vi "HttpGet.vi"(6 "request specific headers":T1[](array[typedef]), 8 "error in":errorcluster, 10 "url":string, 11 "reQwestClient in":refnum<class "reQwestClient.lvclass">) -> (0 "error out":errorcluster, 1 "headers":cluster{"name":string, "value":string}[](array[cluster]), 2 "response_body":string, 3 "reQwestClient out":refnum<class "reQwestClient.lvclass">)   [LabVIEW 2020, in "reQwestClient.lvclass"]
uses:
  reQwestClient.lvclass
  <vilib>/addons/_JKI.lib/REST Client/classes/REST Client/HTTP Header.ctl
  submodules/reqwest-rs-labview/lv_src/Types/http_method_enum.ctl
  reQwestClient.lvclass/reQwestClient.ctl
  submodules/reqwest-rs-labview/lv_src/Request/Request.lvclass
  submodules/reqwest-rs-labview/lv_src/Client/Client.lvclass
  submodules/reqwest-rs-labview/lv_src/reqwest.lvlib
  submodules/reqwest-rs-labview/lv_src/RequestBuilder/RequestBuilder.lvclass
  submodules/reqwest-rs-labview/lv_src/Headers/Headers.lvclass
  <vilib>/addons/_JKI.lib/REST Client/classes/REST Client/REST Client.lvclass
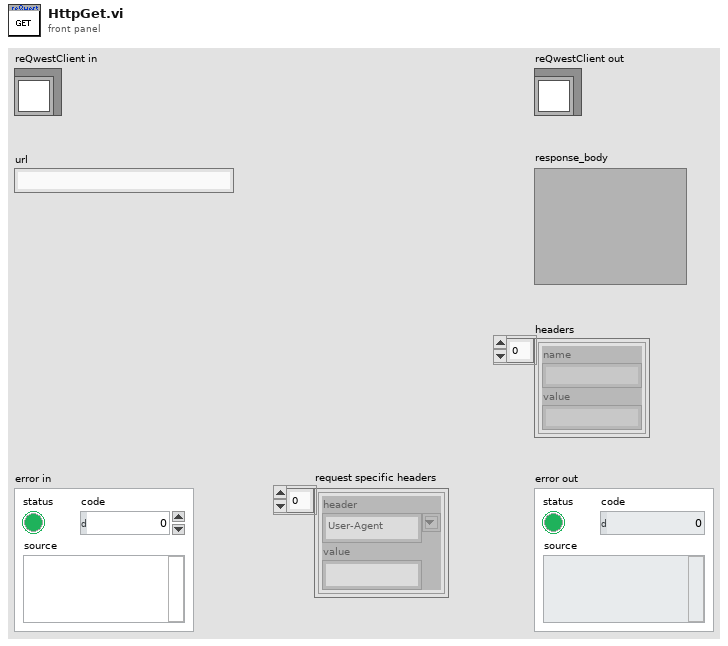
[diagram p1: front panel]
types:
  T1 = typedef "REST Client.lvlib/REST Client.lvclass/HTTP Header.ctl" = cluster{"header":string, "value":string}
  T2 = typedef "reqwest.lvlib/http_method_enum.ctl" = enum8{"<select>", "GET", "POST", "PUT", "DELETE", "HEAD", "OPTIONS", "CONNECT", "PATCH", "TRACE"}
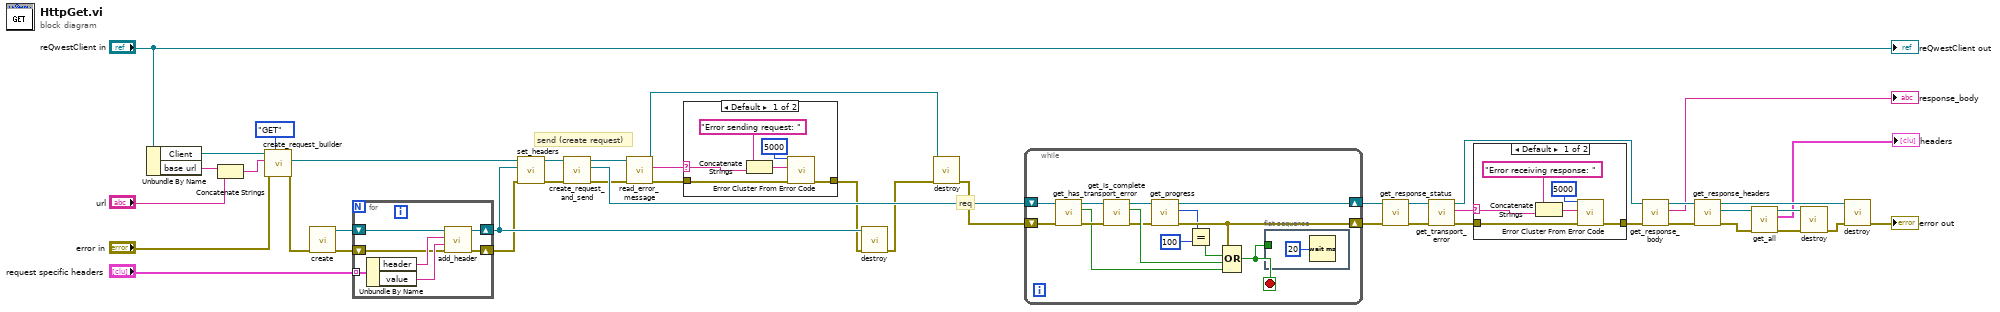
[diagram p0: block diagram]
diagram:
  # "send (create request)"
  # "req"
  n1 = Unbundle By Name("reQwestClient in") -> ("Client"=w25:refnum<class "Client.lvclass">, "base url"=w11:string)
  n2 = Concatenate Strings(w11, "url") -> (w9:string)
  n3 = call "create_request_builder.vi"("HTTP Method"=http_method_enum."GET", "error in (no error)"="error in", "url"=w9, "Client in"=w25) -> ("error out"=w15:errorcluster, "RequestBuilder out"=w21:refnum<class "RequestBuilder.lvclass">)  [unwired: 5 in, 1 out]
  n4 = call "create.vi"("error in (no error)"=w15) -> ("error out"=w22:errorcluster, "Headers out"=w24:refnum<class "Headers.lvclass">)  [unwired: 9 in]
  n5 = for {
    tunnel: "request specific headers" -> [w50] mode=indexing
    shift-right: [w46] -> w18
    shift-left: w24 -> [w51]
    shift-right: [w45] -> w16
    shift-left: w22 -> [w47]
    n6 = Unbundle By Name(w50) -> ("header"=w49:string, "value"=w48:string)
    n7 = call "add_header.vi"("error in (no error)"=w47, "value"=w48, "key"=w49, "Headers in"=w51) -> ("error out"=w45:errorcluster, "Headers out"=w46:refnum<class "Headers.lvclass">)  [unwired: 5 in, 1 out]
  }
  n8 = call "set_headers.vi"("error in (no error)"=w16, "Headers"=w18, "obj in"=w21) -> ("error out"=w19:errorcluster, "obj out"=w20:refnum<class "RequestBuilder.lvclass">)  [unwired: 6 in, 1 out]
  n9 = call "create_request_and_send.vi"("error in"=w19, "obj in"=w20) -> ("error out"=w28:errorcluster, "request"=w31:refnum<class "Request.lvclass">, "obj out"=w29:refnum<class "RequestBuilder.lvclass">)  [unwired: 7 in]
  n10 = call "read_error_message.vi"("error in (no error)"=w28, "RequestBuilder in"=w29) -> ("error out"=w8:errorcluster, "error_message"=w6:string, "RequestBuilder in"=w30:refnum<class "RequestBuilder.lvclass">)  [unwired: 7 in]
  n11 = case shown="Default" w6 {
    selector: w6 -> [w54 _]
    tunnel: w8 -> [w57 w58]
    tunnel: [w56 w58] -> w7
    frame Default {
      n12 = Concatenate Strings("Error sending request: " ("error message (\"\")"), w54) -> (w55:string)
      n13 = call <vilib>:"Error Cluster From Error Code.vi"("error in (no error)"=w57, "error message (\"\")"=w55, "error code (0)"=5000) -> ("error out"=w56:errorcluster)  [unwired: 6 in]
    }
    frame "" {
    }
  }
  n14 = call "destroy.vi"("error in (no error)"=w7, "Headers in"=w18) -> ("error out"=w17:errorcluster)  [unwired: 9 in]
  n15 = call "destroy.vi"("error in"=w17, "RequestBuilder in"=w30) -> ("error out"=w27:errorcluster)  [unwired: 8 in, 1 out]
  n16 = while {
    shift-right: [w70] -> w35
    shift-left: w31 -> [w63]
    shift-right: [w68] -> w34
    shift-left: w27 -> [w62]
    stop <- w64 stop-if-true
    n17 = call "get_has_transport_error.vi"("error in (no error)"=w62, "Request in"=w63) -> ("error out"=w60:errorcluster, "has_transport_error"=w59:bool, "Request out"=w61:refnum<class "Request.lvclass">)  [unwired: 7 in]
    n18 = call "get_is_complete.vi"("error in (no error)"=w60, "Request in"=w61) -> ("error out"=w69:errorcluster, "is_complete"=w72:bool, "Request out"=w71:refnum<class "Request.lvclass">)  [unwired: 7 in]
    n19 = call "get_progress.vi"("error in (no error)"=w69, "Request in"=w71) -> ("error out"=w68:errorcluster, "progress"=w66:i32, "Request out"=w70:refnum<class "Request.lvclass">)  [unwired: 7 in]
    n20 = Equal?(x=w66, y=100 ("progress")) -> (x = y?=w65:bool)
    n21 = Compound Arithmetic op=OR(w68, w65, w72, w59) -> (w64:bool)
    n22 = flat-sequence {
      tunnel: w64 -> [_]
      frame #0 {
        n23 = Wait (ms)(milliseconds to wait=u32 20) -> ()  [unwired: 1 out]
      }
    }
  }
  n24 = call "get_response_status.vi"("error in (no error)"=w34, "Request in"=w35) -> ("error out"=w33:errorcluster, "Request out"=w32:refnum<class "Request.lvclass">)  [unwired: 7 in, 1 out]
  n25 = call "get_transport_error.vi"("error in (no error)"=w33, "Request in"=w32) -> ("error out"=w4:errorcluster, "transport_error"=w5:string, "Request in"=w2:refnum<class "Request.lvclass">)  [unwired: 7 in]
  n26 = case shown="Default" w5 {
    selector: w5 -> [w76 _]
    tunnel: w4 -> [w79 w80]
    tunnel: [w78 w80] -> w3
    frame Default {
      n27 = Concatenate Strings("Error receiving response: " ("error message (\"\")"), w76) -> (w77:string)
      n28 = call <vilib>:"Error Cluster From Error Code.vi"("error in (no error)"=w79, "error message (\"\")"=w77, "error code (0)"=5000) -> ("error out"=w78:errorcluster)  [unwired: 6 in]
    }
    frame "" {
    }
  }
  n29 = call "get_response_body.vi"("error in (no error)"=w3, "Request in"=w2) -> ("error out"=w41:errorcluster, "string_value"=→"response_body":string, "Request in"=w43:refnum<class "Request.lvclass">)  [unwired: 7 in]
  n30 = call "get_response_headers.vi"("error in (no error)"=w41, "Request in"=w43) -> ("error out"=w39:errorcluster, "response_headers"=w40:refnum<class "Headers.lvclass">, "Request in"=w42:refnum<class "Request.lvclass">)  [unwired: 7 in]
  n31 = call "get_all.vi"("error in (no error)"=w39, "Headers in"=w40) -> ("error out"=w37:errorcluster, "headers"=→"headers":cluster{"name":string, "value":string}[], "Headers in"=w38:refnum<class "Headers.lvclass">)  [unwired: 6 in, 1 out]
  n32 = call "destroy.vi"("error in (no error)"=w37, "Headers in"=w38) -> ("error out"=w36:errorcluster)  [unwired: 9 in]
  n33 = call "destroy.vi"("error in (no error)"=w36, "Request in"=w42) -> ("error out"=→"error out":errorcluster)  [unwired: 8 in, 1 out]
  "reQwestClient out" <- "reQwestClient in"
